vi "array index series feb 11 2016 b.vi"() -> ()   [LabVIEW 2015]
panel:
  in  "Array 3":dbl[][](array[numeric])
  out "Boolean 2":bool
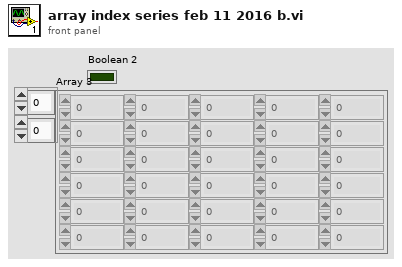
[diagram p1: front panel]
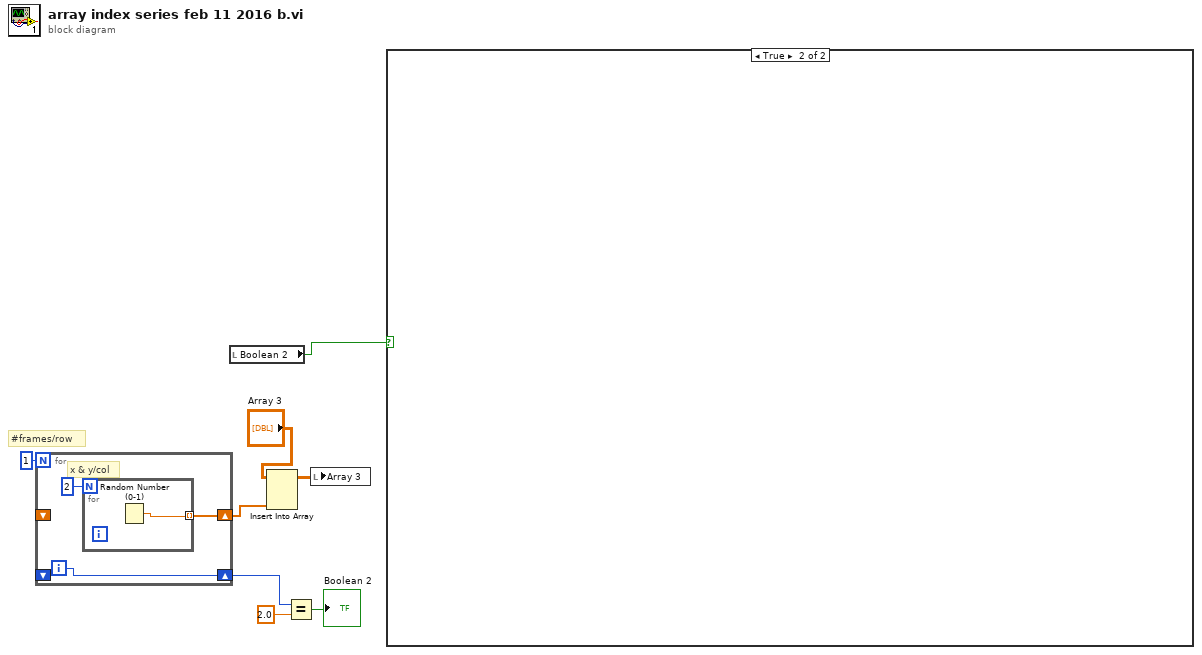
[diagram p0: block diagram]
diagram:
  # "#frames/row"
  n1 = for {
    N: 1 -> [_]
    shift-right: [w9] -> w4
    shift-left: _ -> [_]
    shift-right: [w11] -> w3
    shift-left: _ -> [_]
    i -> [w9]
    # "x & y/col"
    n2 = for {
      N: 2 -> [_]
      tunnel: [w12] -> w11 mode=indexing
      n3 = Random Number (0-1)() -> (number: 0 to 1=w12:dbl)
    }
  }
  n4 = local read "Boolean 2"() -> (w7:bool)
  n5 = Insert Into Array(array="Array 3", new element=w3) -> (w1:dbl[][])  [unwired: 2 in]
  n6 = Equal?(x=w4, y=2.0) -> (x = y?=→"Boolean 2":bool)
  n7 = local write "Array 3"(w1) -> ()
  n8 = case shown="True" w7 {
    frame False {
    }
    frame True {
    }
  }
